vi "ReadVoltage.vi"(8 "error in (no error)":errorcluster, 11 "reference in":refnum<class "VdPhilipsMM-123.lvclass">) -> (0 "error out":errorcluster, 2 "Voltage":dbl, 3 "reference in":refnum<class "VdPhilipsMM-123.lvclass">)   [LabVIEW 2020, in "MulitMeters.lvlib" / "VdPhilipsMM-123.lvclass"]
uses:
  VdPhilipsMM-123.lvclass
  VdPhilipsMM-123.lvclass/VdPhilipsMM-123.ctl
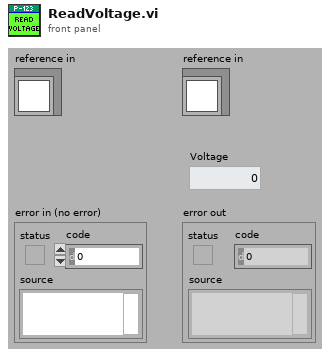
[diagram p1: front panel]
types:
  T1 = typedef "MulitMeters.lvlib/VdPhilipsMM-123.lvclass/ObjectAttributes.ctl" = cluster{"Attribute1":dbl}
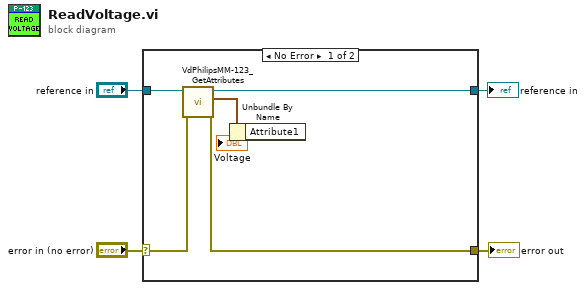
[diagram p0: block diagram]
diagram:
  n1 = case shown="No Error" "error in (no error)" {
    selector: "error in (no error)" -> [w9 w11]
    tunnel: [w7 w11] -> w3
    tunnel: [w5 w10] -> w1
    tunnel: "reference in" -> [w6 w10]
    frame No Error {
      n2 = call "VdPhilipsMM-123_GetAttributes.vi"("error in (no error)"=w9, "reference in"=w6) -> ("error out"=w7:errorcluster, "Data"=w8:T1, "reference out"=w5:refnum<class "VdPhilipsMM-123.lvclass">)  [unwired: 6 in, 1 out]
      n3 = Unbundle By Name(w8) -> ()  [unwired: 1 out]
    }
    frame Error {
    }
  }
  "error out" <- w3
  "reference in" <- w1
